vi "Main.vi"() -> ()   [LabVIEW 2016]
uses:
  Message Format.ctl
  Queue Cluster.ctl
  StateDef_generic.ctl
panel:
  in  "Enable":bool
  in  "Target":dbl
  in  "Log":bool
  in  "Pitchpack_Home":bool
  in  "Pitchpack_Stop":bool
  in  "PitchPack_Move":bool
  in  "Exit":bool
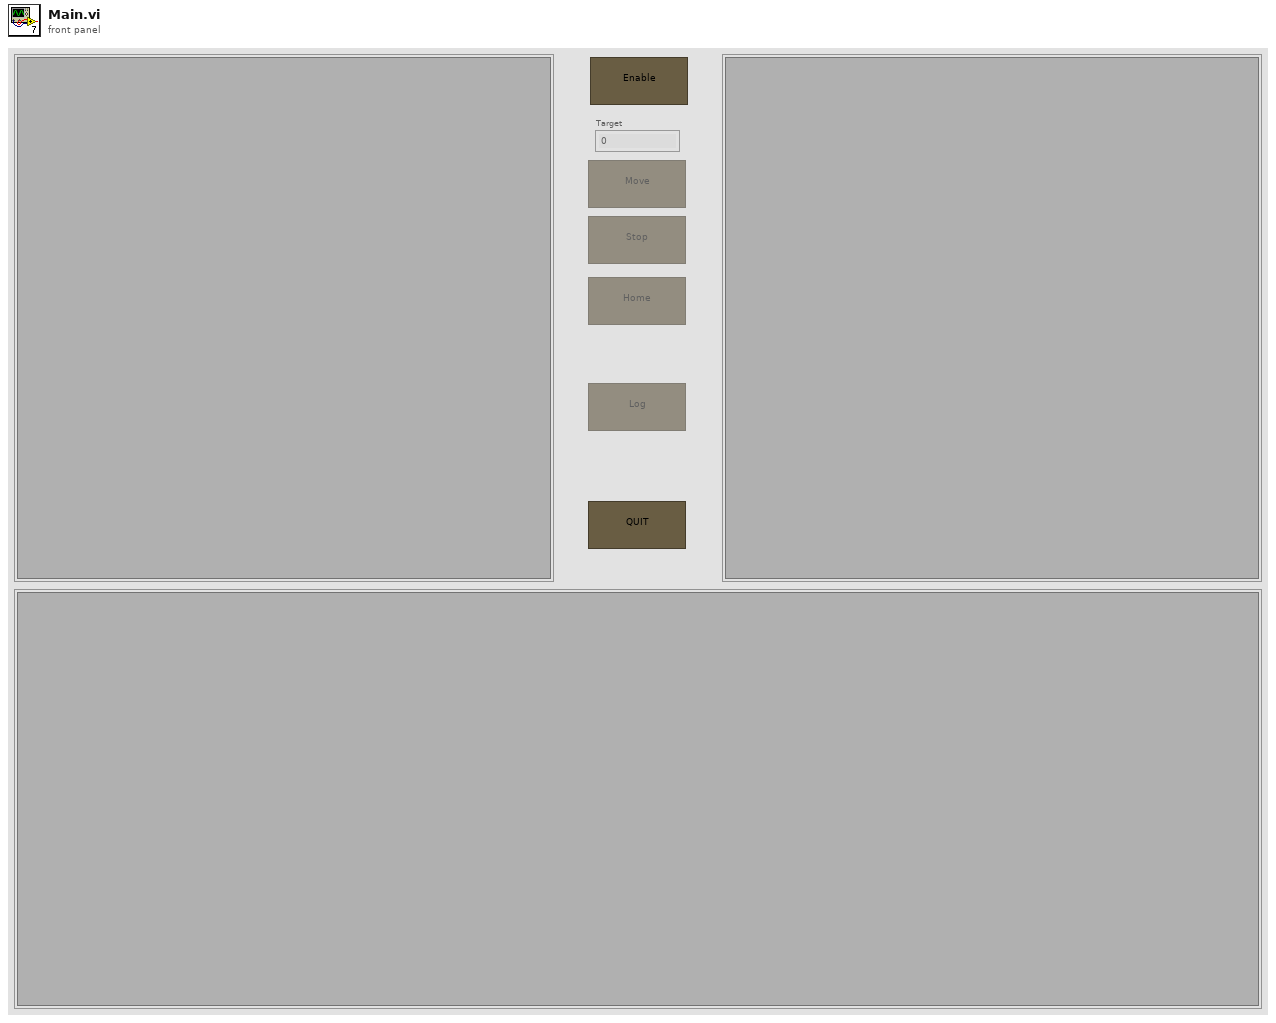
[diagram p1: front panel]
types:
  T1 = typedef "StateDef_generic.ctl" = enum16{"Initialize", "Running", "Exit"}
  T2 = typedef "Message Format.ctl" = cluster{"header":string, "data":variant}
  T3 = typedef "Queue Cluster.ctl" = cluster{"GUI":refnum<queue>, "Logger":refnum<queue>, "Pipeline":refnum<queue>, "ExternalData":refnum<queue>, "VehicleData":refnum<queue>, "VibrationData":refnum<queue>, "Receive":refnum<queue>, "Transmit":refnum<queue>}
  T4 = enum8{"Enabled", "Disabled", "Disabled and Grayed Out"}
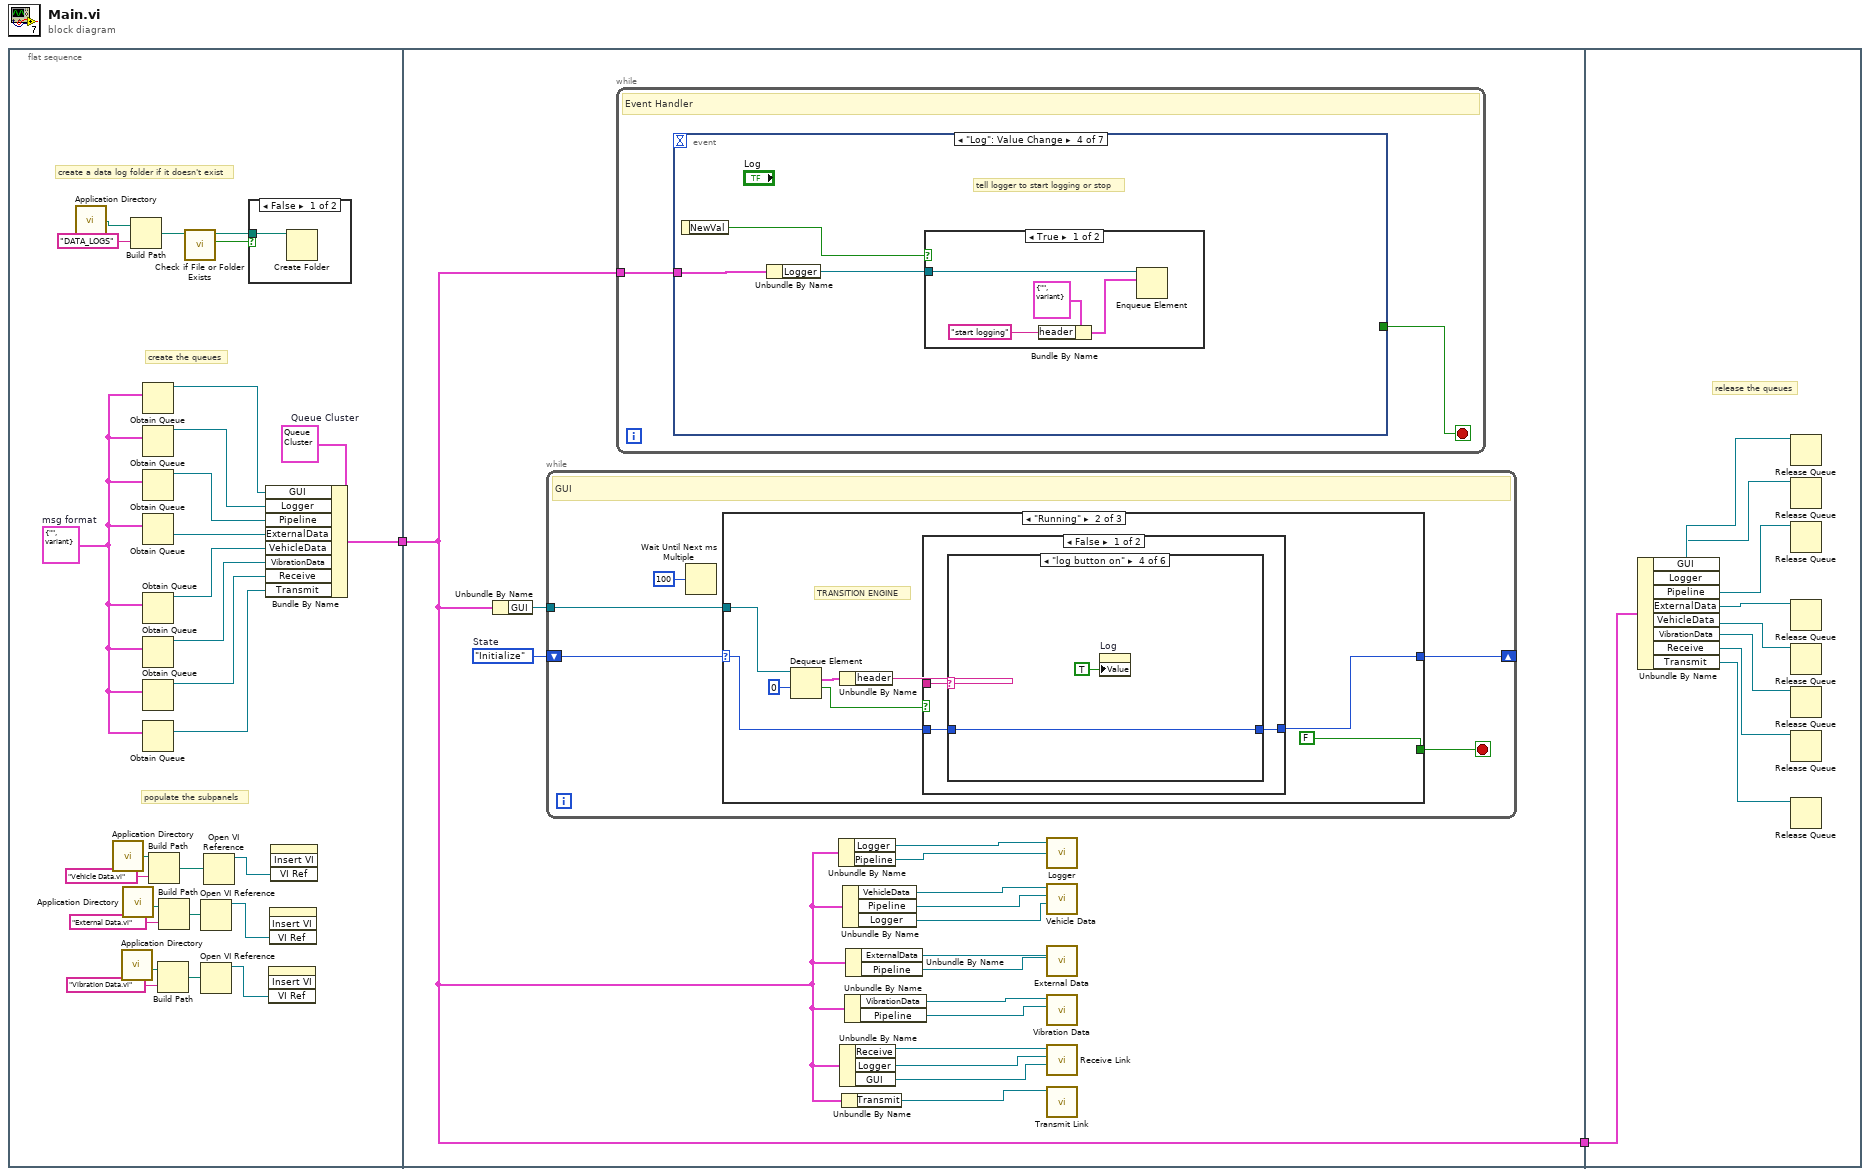
[diagram p0: block diagram]
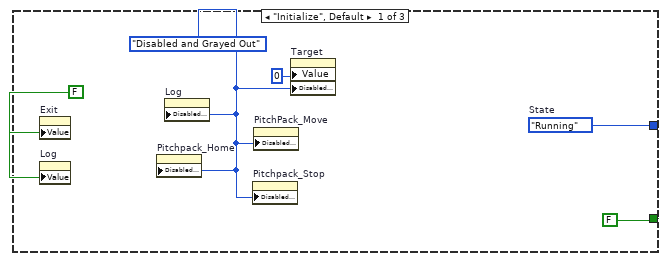
[diagram p3: hidden frame]
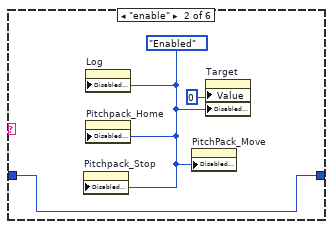
[diagram p5: hidden frame]
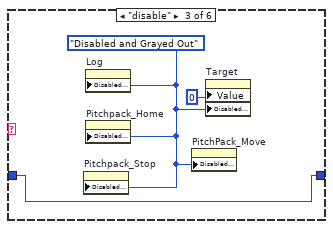
[diagram p6: hidden frame]
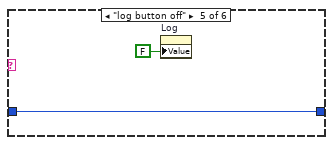
[diagram p7: hidden frame]
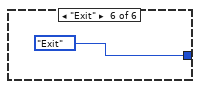
[diagram p8: hidden frame]
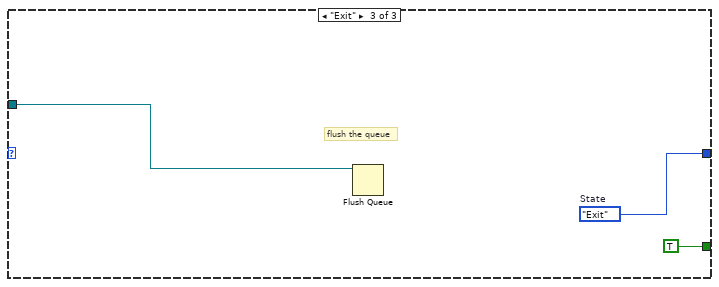
[diagram p10: hidden frame]
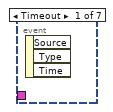
[diagram p11: hidden frame]
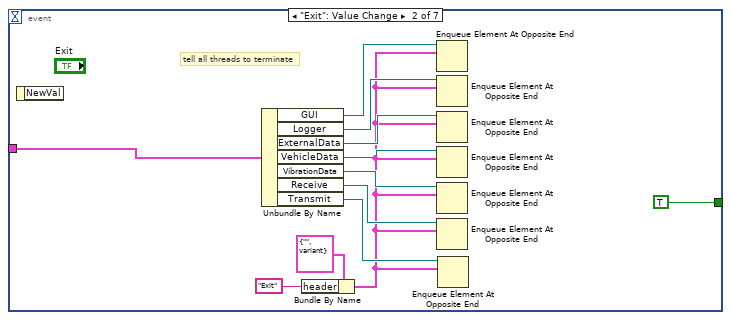
[diagram p12: hidden frame]
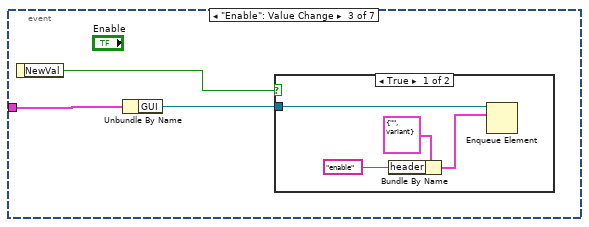
[diagram p13: hidden frame]
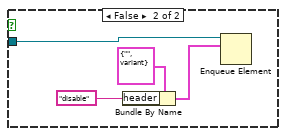
[diagram p14: hidden frame]
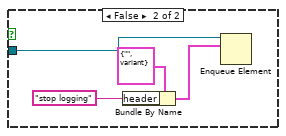
[diagram p15: hidden frame]
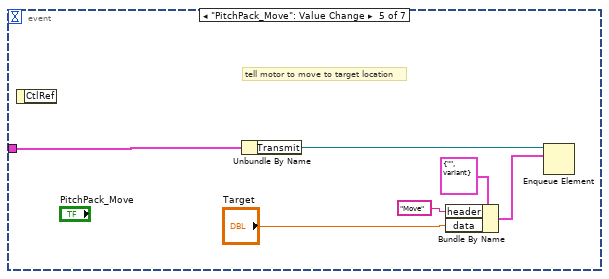
[diagram p16: hidden frame]
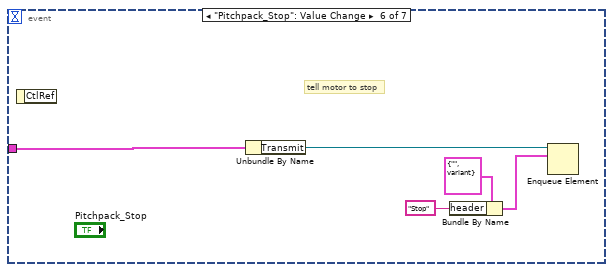
[diagram p17: hidden frame]
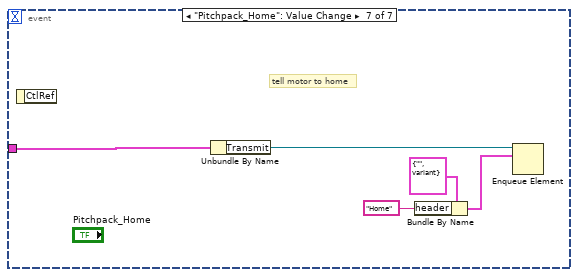
[diagram p18: hidden frame]
diagram:
  n1 = flat-sequence {
    tunnel: [w17] -> w2
    tunnel: w2 -> [w33]
    tunnel: [w33] -> w1
    tunnel: w1 -> [w145]
    frame #0 {
      w18 = T3 {"GUI"=refnum, "Logger"=refnum, "Pipeline"=refnum, "ExternalData"=refnum, "VehicleData"=refnum, "VibrationData"=refnum, "Receive"=refnum, "Transmit"=refnum}  # Queue Cluster
      w4 = T2 {"header"="", "data"=variant}  # msg format
      # "populate the subpanels"
      # "create the queues"
      # "create a data log folder if it doesn't exist"
      n2 = call <vilib>:"Application Directory.vi"() -> ("Application Directory"=w28:path)
      n3 = call <vilib>:"Application Directory.vi"() -> ("Application Directory"=w8:path)
      n4 = call <vilib>:"Application Directory.vi"() -> ("Application Directory"=w14:path)
      n5 = call <vilib>:"Application Directory.vi"() -> ("Application Directory"=w12:path)
      n6 = Build Path(base path=w28, name or relative path="DATA_LOGS") -> (appended path=w26:path)
      n7 = Obtain Queue(element data type=w4) -> (queue out=w19:refnum<queue>)  [unwired: 4 in, 2 out]
      n8 = Obtain Queue(element data type=w4) -> (queue out=w20:refnum<queue>)  [unwired: 4 in, 2 out]
      n9 = Obtain Queue(element data type=w4) -> (queue out=w21:refnum<queue>)  [unwired: 4 in, 2 out]
      n10 = Obtain Queue(element data type=w4) -> (queue out=w22:refnum<queue>)  [unwired: 4 in, 2 out]
      n11 = Obtain Queue(element data type=w4) -> (queue out=w23:refnum<queue>)  [unwired: 4 in, 2 out]
      n12 = Obtain Queue(element data type=w4) -> (queue out=w24:refnum<queue>)  [unwired: 4 in, 2 out]
      n13 = Obtain Queue(element data type=w4) -> (queue out=w25:refnum<queue>)  [unwired: 4 in, 2 out]
      n14 = Obtain Queue(element data type=w4) -> (queue out=w3:refnum<queue>)  [unwired: 4 in, 2 out]
      n15 = Build Path(base path=w8, name or relative path="Vehicle Data.vi") -> (appended path=w10:path)
      n16 = Build Path(base path=w14, name or relative path="Vibration Data.vi") -> (appended path=w16:path)
      n17 = Build Path(base path=w12, name or relative path="External Data.vi") -> (appended path=w13:path)
      n18 = call <vilib>:"Check if File or Folder Exists.vi"("path"=w26) -> ("file or folder exists?"=w29:bool, "dup path"=w30:path)  [unwired: 8 in, 1 out]
      n19 = Open VI Reference(vi path=w13) -> (vi reference=w6:refnum<vi>)  [unwired: 5 in, 1 out]
      n20 = Open VI Reference(vi path=w16) -> (vi reference=w7:refnum<vi>)  [unwired: 5 in, 1 out]
      n21 = Open VI Reference(vi path=w10) -> (vi reference=w5:refnum<vi>)  [unwired: 5 in, 1 out]
      n22 = case shown="False" w29 {
        tunnel: w30 -> [w31 _]
        frame False {
          n23 = Create Folder(path (use dialog)=w31) -> ()  [unwired: 2 in, 3 out]
        }
        frame True {
        }
      }
      n24 = Bundle By Name(cluster=w18, "GUI"=w19, "Logger"=w20, "Pipeline"=w21, "ExternalData"=w22, "VehicleData"=w23, "VibrationData"=w24, "Receive"=w25, "Transmit"=w3) -> (w17:T3)
      n25 = invoke on="Sub Panel" class="SubPnl" method="Insert VI"("VI Ref"=w7) -> ()  [unwired: 3 in, 4 out]
      n26 = invoke on="Sub Panel" class="SubPnl" method="Insert VI"("VI Ref"=w6) -> ()  [unwired: 3 in, 4 out]
      n27 = invoke on="Sub Panel" class="SubPnl" method="Insert VI"("VI Ref"=w5) -> ()  [unwired: 3 in, 4 out]
    }
    frame #1 {
      w40 = StateDef_generic."Initialize"  # State
      n28 = Unbundle By Name(w33) -> ("GUI"=w41:refnum<queue>)
      n29 = while {
        tunnel: w41 -> [w48]
        shift-right: [w49] -> _
        shift-left: w40 -> [w50]
        stop <- w51 stop-if-true
        # "GUI"
        n30 = Wait Until Next ms Multiple(millisecond multiple=u32 100) -> ()  [unwired: 1 out]
        n31 = case shown="\"Running\"" w50 {
          selector: w50 -> [_ w59 _]
          tunnel: [FALSE FALSE TRUE] -> w51
          tunnel: [w55 w60 w83] -> w49
          tunnel: w48 -> [_ w61 w82]
          frame "Initialize", Default {
            w53 = T4."Disabled and Grayed Out" ("Disabled")
            w55 = StateDef_generic."Running"  # State
            w57 = FALSE ("Connect")
            n32 = property on="Exit" class="Bool (strict)"("Value"=w57) -> ()  [unwired: 2 in, 2 out]
            n33 = property on="Log" class="Bool (strict)"("Value"=w57) -> ()  [unwired: 2 in, 2 out]
            n34 = property on="Pitchpack_Home" class="Bool"("DisabledEnum"=w53) -> ()  [unwired: 2 in, 2 out]
            n35 = property on="Log" class="Bool (strict)"("DisabledEnum"=w53) -> ()  [unwired: 2 in, 2 out]
            n36 = property on="Pitchpack_Stop" class="Bool"("DisabledEnum"=w53) -> ()  [unwired: 2 in, 2 out]
            n37 = property on="PitchPack_Move" class="Bool"("DisabledEnum"=w53) -> ()  [unwired: 2 in, 2 out]
            n38 = property on="Target" class="DigNum (strict)"("Value"=0 ("Target"), "DisabledEnum"=w53) -> ()  [unwired: 2 in, 2 out]
          }
          frame "Running" {
            # "TRANSITION ENGINE"
            n39 = Dequeue Element(queue=w61, timeout in ms (-1)=0) -> (element=w64:T2, timed out?=w62:bool)  [unwired: 1 in, 2 out]
            n40 = Unbundle By Name(w64) -> ("header"=w63:string)
            n41 = case shown="False" w62 {
              tunnel: w63 -> [w68 _]
              tunnel: [w67 w81] -> w60
              tunnel: w59 -> [w66 w81]
              frame False {
                n42 = case shown="\"log button on\"" w68 {
                  tunnel: [w69 w70 w73 w76 w78 StateDef_generic."Exit" ("State")] -> w67
                  tunnel: w66 -> [w69 w70 w73 w76 w78 _]
                  frame "any other", Default {
                  }
                  frame "enable" {
                    w71 = T4."Enabled" ("Disabled")
                    n43 = property on="Pitchpack_Stop" class="Bool"("DisabledEnum"=w71) -> ()  [unwired: 2 in, 2 out]
                    n44 = property on="Log" class="Bool (strict)"("DisabledEnum"=w71) -> ()  [unwired: 2 in, 2 out]
                    n45 = property on="Pitchpack_Home" class="Bool"("DisabledEnum"=w71) -> ()  [unwired: 2 in, 2 out]
                    n46 = property on="PitchPack_Move" class="Bool"("DisabledEnum"=w71) -> ()  [unwired: 2 in, 2 out]
                    n47 = property on="Target" class="DigNum (strict)"("Value"=0 ("Target"), "DisabledEnum"=w71) -> ()  [unwired: 2 in, 2 out]
                  }
                  frame "disable" {
                    w74 = T4."Disabled and Grayed Out" ("Disabled")
                    n48 = property on="Pitchpack_Stop" class="Bool"("DisabledEnum"=w74) -> ()  [unwired: 2 in, 2 out]
                    n49 = property on="Log" class="Bool (strict)"("DisabledEnum"=w74) -> ()  [unwired: 2 in, 2 out]
                    n50 = property on="Pitchpack_Home" class="Bool"("DisabledEnum"=w74) -> ()  [unwired: 2 in, 2 out]
                    n51 = property on="PitchPack_Move" class="Bool"("DisabledEnum"=w74) -> ()  [unwired: 2 in, 2 out]
                    n52 = property on="Target" class="DigNum (strict)"("Value"=0 ("Target"), "DisabledEnum"=w74) -> ()  [unwired: 2 in, 2 out]
                  }
                  frame "log button on" {
                    n53 = property on="Log" class="Bool (strict)"("Value"=TRUE ("Log")) -> ()  [unwired: 2 in, 2 out]
                  }
                  frame "log button off" {
                    n54 = property on="Log" class="Bool (strict)"("Value"=FALSE ("Log")) -> ()  [unwired: 2 in, 2 out]
                  }
                  frame "Exit" {
                  }
                }
              }
              frame True {
              }
            }
          }
          frame "Exit" {
            w83 = StateDef_generic."Exit"  # State
            # "flush the queue"
            n55 = Flush Queue(queue=w82) -> ()  [unwired: 1 in, 3 out]
          }
        }
      }
      n56 = while {
        tunnel: w33 -> [w85]
        stop <- w86 stop-if-true
        # "Event Handler"
        n57 = event shown="[3] \"Log\": Value Change" {
          selector: _ -> [_ _ _ _ _ _ _]
          dyn-events: _ -> [_ _ _ _ _ _ _]
          timeout: _ -> [_ _ _ _ _ _ _]
          tunnel: [_ TRUE ("User Event") _ _ _ _ _] -> w86
          tunnel: w85 -> [_ w89 w99 w111 w123 w128 w132]
          event Timeout {
            n58 = event-data() -> ()  [unwired: 1 in, 3 out]
          }
          event "Exit": Value Change {
            # "tell all threads to terminate"
            n59 = event-data() -> ()  [unwired: 1 in, 1 out]
            n60 = Unbundle By Name(w89) -> ("GUI"=w95:refnum<queue>, "Logger"=w94:refnum<queue>, "ExternalData"=w93:refnum<queue>, "VehicleData"=w92:refnum<queue>, "VibrationData"=w91:refnum<queue>, "Receive"=w90:refnum<queue>, "Transmit"=w88:refnum<queue>)
            n61 = Bundle By Name(cluster=T2 {"header"="", "data"=variant} ("msg format"), "header"="Exit") -> (w87:T2)
            n62 = Enqueue Element At Opposite End(queue=w95, element=w87) -> ()  [unwired: 2 in, 3 out]
            n63 = Enqueue Element At Opposite End(queue=w94, element=w87) -> ()  [unwired: 2 in, 3 out]
            n64 = Enqueue Element At Opposite End(queue=w93, element=w87) -> ()  [unwired: 2 in, 3 out]
            n65 = Enqueue Element At Opposite End(queue=w92, element=w87) -> ()  [unwired: 2 in, 3 out]
            n66 = Enqueue Element At Opposite End(queue=w91, element=w87) -> ()  [unwired: 2 in, 3 out]
            n67 = Enqueue Element At Opposite End(queue=w90, element=w87) -> ()  [unwired: 2 in, 3 out]
            n68 = Enqueue Element At Opposite End(queue=w88, element=w87) -> ()  [unwired: 2 in, 3 out]
          }
          event "Enable": Value Change {
            n69 = event-data() -> ("NewVal"=w100:bool)  [unwired: 1 in]
            n70 = Unbundle By Name(w99) -> ("GUI"=w101:refnum<queue>)
            n71 = case shown="True" w100 {
              tunnel: w101 -> [w102 w106]
              frame True {
                n72 = Bundle By Name(cluster=T2 {"header"="", "data"=variant} ("msg format"), "header"="enable") -> (w103:T2)
                n73 = Enqueue Element(queue=w102, element=w103) -> ()  [unwired: 2 in, 3 out]
              }
              frame False {
                n74 = Bundle By Name(cluster=T2 {"header"="", "data"=variant} ("msg format"), "header"="disable") -> (w107:T2)
                n75 = Enqueue Element(queue=w106, element=w107) -> ()  [unwired: 2 in, 3 out]
              }
            }
          }
          event "Log": Value Change {
            # "tell logger to start logging or stop"
            n76 = event-data() -> ("NewVal"=w112:bool)  [unwired: 1 in]
            n77 = Unbundle By Name(w111) -> ("Logger"=w110:refnum<queue>)
            n78 = case shown="True" w112 {
              tunnel: w110 -> [w113 w117]
              frame True {
                n79 = Bundle By Name(cluster=T2 {"header"="", "data"=variant} ("msg format"), "header"="start logging") -> (w114:T2)
                n80 = Enqueue Element(queue=w113, element=w114) -> ()  [unwired: 2 in, 3 out]
              }
              frame False {
                n81 = Bundle By Name(cluster=T2 {"header"="", "data"=variant} ("msg format"), "header"="stop logging") -> (w118:T2)
                n82 = Enqueue Element(queue=w117, element=w118) -> ()  [unwired: 2 in, 3 out]
              }
            }
          }
          event "PitchPack_Move": Value Change {
            # "tell motor to move to target location"
            n83 = event-data() -> ()  [unwired: 1 in, 1 out]
            n84 = Unbundle By Name(w123) -> ("Transmit"=w122:refnum<queue>)
            n85 = Bundle By Name(cluster=T2 {"header"="", "data"=variant} ("msg format"), "header"="Move", "data"="Target") -> (w124:T2)
            n86 = Enqueue Element(queue=w122, element=w124) -> ()  [unwired: 2 in, 3 out]
          }
          event "Pitchpack_Stop": Value Change {
            # "tell motor to stop"
            n87 = event-data() -> ()  [unwired: 1 in, 1 out]
            n88 = Unbundle By Name(w128) -> ("Transmit"=w127:refnum<queue>)
            n89 = Bundle By Name(cluster=T2 {"header"="", "data"=variant} ("msg format"), "header"="Stop") -> (w129:T2)
            n90 = Enqueue Element(queue=w127, element=w129) -> ()  [unwired: 2 in, 3 out]
          }
          event "Pitchpack_Home": Value Change {
            # "tell motor to home"
            n91 = event-data() -> ()  [unwired: 1 in, 1 out]
            n92 = Unbundle By Name(w132) -> ("Transmit"=w133:refnum<queue>)
            n93 = Bundle By Name(cluster=T2 {"header"="", "data"=variant} ("msg format"), "header"="Home") -> (w134:T2)
            n94 = Enqueue Element(queue=w133, element=w134) -> ()  [unwired: 2 in, 3 out]
          }
        }
      }
      n95 = Unbundle By Name(w33) -> ("Logger"=w38:refnum<queue>, "Pipeline"=w37:refnum<queue>)
      n96 = Unbundle By Name(w33) -> ("Receive"=w39:refnum<queue>, "Logger"=w35:refnum<queue>, "GUI"=w32:refnum<queue>)
      n97 = Unbundle By Name(w33) -> ("Transmit"=w34:refnum<queue>)
      n98 = Unbundle By Name(w33) -> ("VehicleData"=w45:refnum<queue>, "Pipeline"=w42:refnum<queue>, "Logger"=w36:refnum<queue>)
      n99 = Unbundle By Name(w33) -> ("VibrationData"=w47:refnum<queue>, "Pipeline"=w44:refnum<queue>)
      n100 = Unbundle By Name(w33) -> ("ExternalData"=w46:refnum<queue>, "Pipeline"=w43:refnum<queue>)
      n101 = call "Logger.vi"("Pipeline In"=w37, "Logger Queue In"=w38) -> ()  [unwired: 3 in, 1 out]
      n102 = call "Vehicle Data.vi"("Logger In"=w36, "Pipeline In"=w42, "Vehicle Queue In"=w45) -> ()  [unwired: 8 in, 1 out]
      n103 = call "External Data.vi"("Pipeline In"=w43, "External Queue In"=w46) -> ()  [unwired: 9 in, 1 out]
      n104 = call "Vibration Data.vi"("Pipeline In"=w44, "Vibration Queue In"=w47) -> ()  [unwired: 9 in, 1 out]
      n105 = call "Receive Link.vi"("GUI Queue In"=w32, "Logger Queue In"=w35, "Receive Queue In"=w39) -> ()  [unwired: 8 in, 1 out]
      n106 = call "Transmit Link.vi"("Transmit Queue In"=w34) -> ()  [unwired: 10 in, 1 out]
    }
    frame #2 {
      # "release the queues"
      n107 = Unbundle By Name(w145) -> ("GUI"=w144:refnum<queue>, "Logger"=w143:refnum<queue>, "Pipeline"=w142:refnum<queue>, "ExternalData"=w138:refnum<queue>, "VehicleData"=w141:refnum<queue>, "VibrationData"=w140:refnum<queue>, "Receive"=w139:refnum<queue>, "Transmit"=w137:refnum<queue>)
      n108 = Release Queue(queue=w144) -> ()  [unwired: 2 in, 3 out]
      n109 = Release Queue(queue=w143) -> ()  [unwired: 2 in, 3 out]
      n110 = Release Queue(queue=w142) -> ()  [unwired: 2 in, 3 out]
      n111 = Release Queue(queue=w138) -> ()  [unwired: 2 in, 3 out]
      n112 = Release Queue(queue=w141) -> ()  [unwired: 2 in, 3 out]
      n113 = Release Queue(queue=w140) -> ()  [unwired: 2 in, 3 out]
      n114 = Release Queue(queue=w139) -> ()  [unwired: 2 in, 3 out]
      n115 = Release Queue(queue=w137) -> ()  [unwired: 2 in, 3 out]
    }
  }
